vi "save_imd3.vi"(0 "Apeak":dbl[](array[numeric]), 1 "Apeakpos":dbl[](array[numeric]), 2 "Apeaknext":dbl[](array[numeric]), 3 "Anextpos":dbl[](array[numeric]), 4 "Bpeak":dbl[](array[numeric]), 5 "Bpeakpos":dbl[](array[numeric]), 6 "PATH":string, 7 "Bpeaknext":dbl[](array[numeric]), 8 "Tabsize":dbl, 9 "Bnextpos":dbl[](array[numeric]), 10 "FreqTab":dbl[](array[numeric]), 11 "RApeak":dbl[](array[numeric]), 13 "RApos":dbl[](array[numeric]), 18 "RBpos":dbl[](array[numeric]), 19 "RBpeak":dbl[](array[numeric])) -> ()   [LabVIEW 2015]
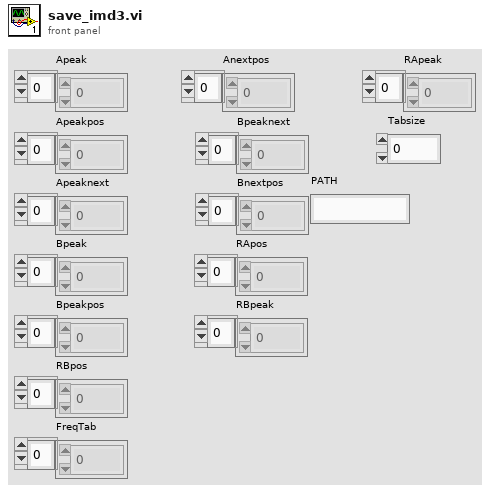
[diagram p1: front panel]
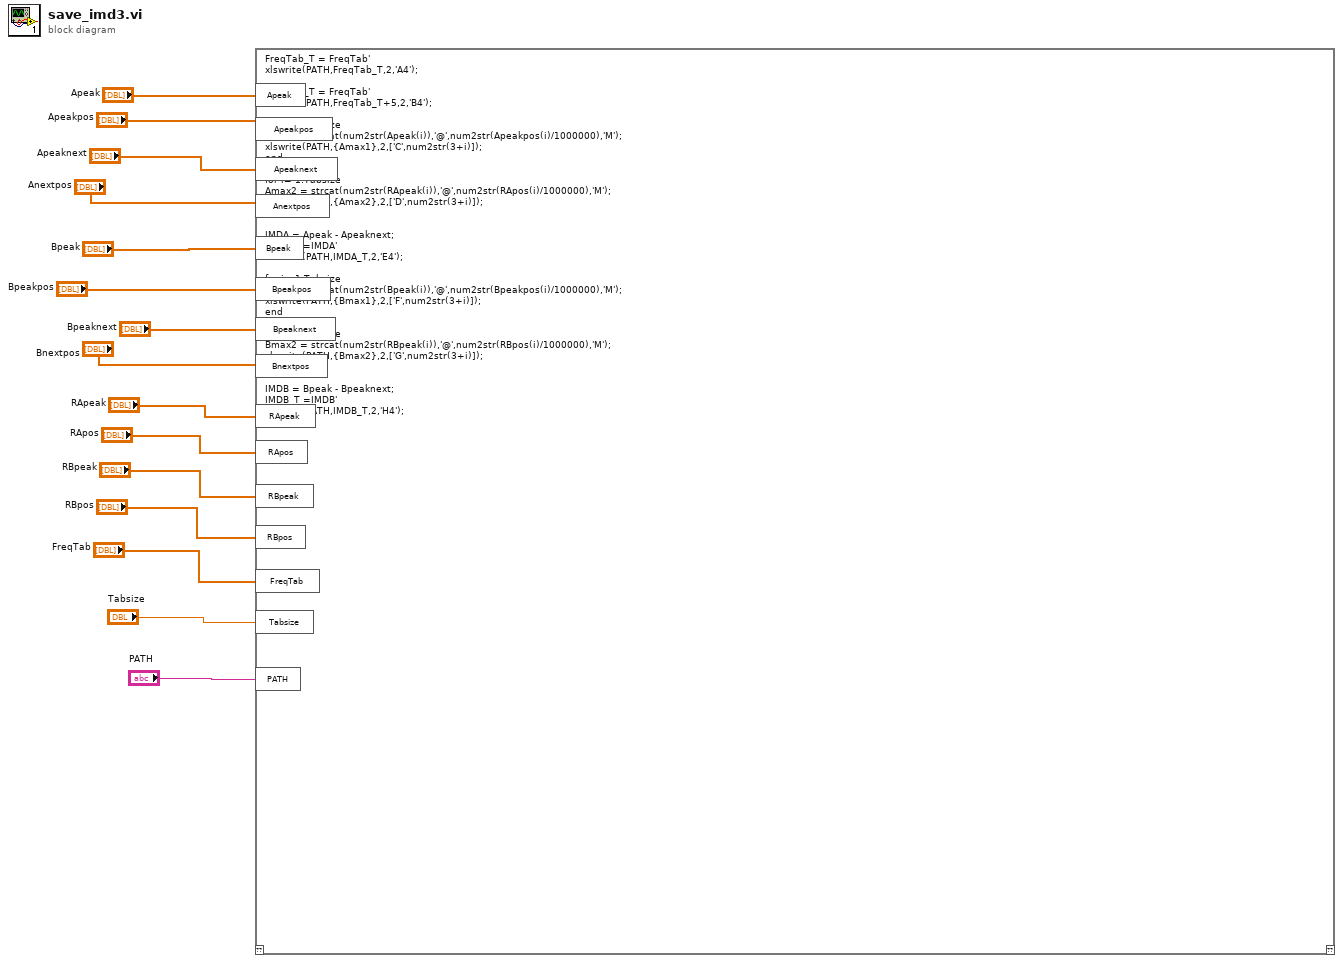
[diagram p0: block diagram]
diagram:
  n1 = script code="FreqTab_T = FreqTab'\nxlswrite(PATH,FreqTab_T,2,'A4');\n\nFreqTab_T = FreqTab'\nxlswrite(PATH,FreqTab_T+5,2,'B4');\n\nfor i= 1:Tabsize\nAmax1 = strcat(num2str(Apeak(i)),'@',num2str(Apeakpos(i)/1000000),'M');\nxlswrite(PATH,{Amax1},2,['C',num2str(3+i)]);\nend\n\nfor i= 1:Tabsize\nAmax2 = strcat(num2str(RApeak(i)),'@',num2str(RApos(i)/1000000),'M');\nxlswrite(PATH,{Amax2},2,['D',num2str(3+i)]);\nend\n\nIMDA = Apeak - Apeaknext;\nIMDA_T =IMDA'\nxlswrite(PATH,IMDA_T,2,'E4');\n\nfor i= 1:Tabsize\nBmax1 = strcat(num2str(Bpeak(i)),'@',num2str(Bpeakpos(i)/1000000),'M');\nxlswrite(PATH,{Bmax1},2,['F',num2str(3+i)]);\nend\n\nfor i= 1:Tabsize\nBmax2 = strcat(num2str(RBpeak(i)),'@',num2str(RBpos(i)/1000000),'M');\nxlswrite(PATH,{Bmax2},2,['G',num2str(3+i)]);\nend\n\nIMDB = Bpeak - Bpeaknext;\nIMDB_T =IMDB'\nxlswrite(PATH,IMDB_T,2,'H4');"("Apeak"="Apeak", "Apeakpos"="Apeakpos", "Apeaknext"="Apeaknext", "Anextpos"="Anextpos", "Bpeak"="Bpeak", "Bpeakpos"="Bpeakpos", "Bpeaknext"="Bpeaknext", "Bnextpos"="Bnextpos", "RApeak"="RApeak", "RApos"="RApos", "RBpeak"="RBpeak", "RBpos"="RBpos", "FreqTab"="FreqTab", "Tabsize"="Tabsize", "PATH"="PATH") -> ()  [unwired: 1 in, 1 out]
